vi "Sequence Get.vi"(8 "error in (no error)":errorcluster, 10 "sxSequenceId (\"\")":string, 11 "Connection Refnum":T1) -> (0 "error out":errorcluster, 2 "Sequence Record":T2, 3 "Connection Refnum":T1, 4 "Data Present":bool)   [LabVIEW 2011]
uses:
  Sequence Record.ctl
  Summitek EXT/ODBC/SQL Controls/Connection Refnum.ctl
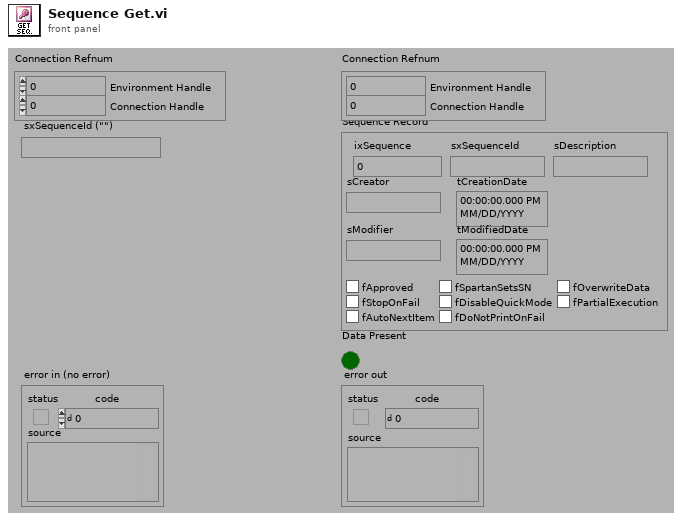
[diagram p1: front panel]
types:
  T1 = typedef "Connection Refnum.ctl" = cluster{"Environment Handle":i32, "Connection Handle":i32}
  T2 = typedef "Sequence Record.ctl" = cluster{"ixSequence":i32, "sxSequenceId":string, "sDescription":string, "sCreator":string, "tCreationDate":timestamp, "sModifier":string, "tModifiedDate":timestamp, "fApproved":bool, "fSpartanSetsSN":bool, "fOverwriteData":bool, "fStopOnFail":bool, "fDisableQuickMode":bool, "fPartialExecution":bool, "fAutoNextItem":bool, "fDoNotPrintOnFail":bool}
  T3 = typedef "Statement Refnum.ctl" = cluster{"Statement Handle":i32, "Parameter Number":u16}
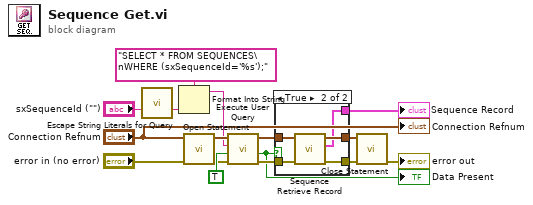
[diagram p0: block diagram]
diagram:
  n1 = call "Escape String Literals for Query.vi"("String"="sxSequenceId (\"\")") -> ("escaped String"=w1:string)  [unwired: 1 in, 13 out]
  n2 = Format Into String(format string="SELECT * FROM SEQUENCES\nWHERE (sxSequenceId='%s');" ("User Query"), w1) -> (resulting string=w8:string)  [unwired: 2 in, 1 out]
  n3 = call "Open Statement.vi"("error in (no error)"="error in (no error)", "Connection Refnum"="Connection Refnum") -> ("error out"=w9:errorcluster, "Statement Refnum"=w10:T3)  [unwired: 4 out]
  n4 = call "Execute User Query.vi"("error in (no error)"=w9, "Return Data? (f)"=TRUE, "User Query"=w8, "Statement Refnum"=w10) -> ("error out"=w16:errorcluster, "Data Present?"=w7:bool, "Statement Refnum"=w15:T3)  [unwired: 1 out]
  "Data Present" <- w7
  n5 = case shown="True" w7 {
    tunnel: w16 -> [w17 w22]
    tunnel: w15 -> [w18 w23]
    tunnel: [w17 w20] -> w12
    tunnel: [w18 w21] -> w13
    tunnel: [_ w19] -> w2
    frame False {
    }
    frame True {
      n6 = call "Sequence Retrieve Record.vi"("error in (no error)"=w22, "Statement Refnum"=w23) -> ("error out"=w20:errorcluster, "Sequence Record"=w19:T2, "Statement Refnum"=w21:T3)  [unwired: 7 out]
    }
  }
  "Sequence Record" <- w2
  n7 = call "Close Statement.vi"("error in (no error)"=w12, "Statement Refnum"=w13) -> ("error out"=→"error out":errorcluster)  [unwired: 5 out]
  "Connection Refnum" <- "Connection Refnum"
